vi "Call Remote Restart Camera server.vi"() -> (0 "Error out":errorcluster)   [LabVIEW 2015]
doc: "Asynchronously gets a snapshot image from the selected camera on the camera server and saves it to the specified path with specified name."
panel:
  # "PN 08/08/16"
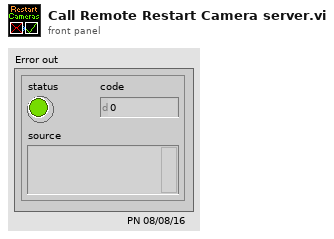
[diagram p1: front panel]
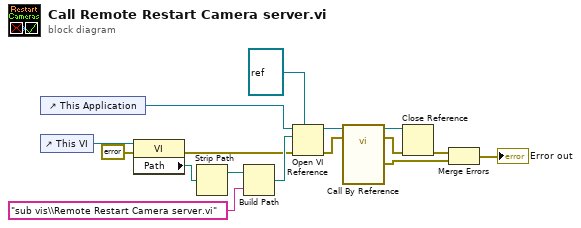
[diagram p0: block diagram]
diagram:
  n1 = control-ref of="This Application"() -> (w11:refnum<vi>)
  n2 = control-ref of="This VI"() -> (w16:refnum<vi>)
  n3 = property class="VI"(reference=w16, error in=errorcluster {"status"=FALSE, "code"=0, "source"=""} ("error in (no error)")) -> (error out=w13:errorcluster, "Path"=w10:path)  [unwired: 1 out]
  n4 = Strip Path(path=w10) -> (stripped path=w9:path)  [unwired: 1 out]
  n5 = Build Path(base path=w9, name or relative path="sub vis\\Remote Restart Camera server.vi") -> (appended path=w14:path)
  n6 = Open VI Reference(type specifier VI Refnum (for type only)=refnum<vi> refnum, application reference (local)=w11, vi path=w14, error in (no error)=w13) -> (vi reference=w8:refnum<vi>, error out=w7:errorcluster)  [unwired: 2 in]
  n7 = call-by-ref "?"(reference=w8, error in=w7) -> (reference out=w3:refnum<vi>, error out=w2:errorcluster, "Error out"=w1:errorcluster)
  n8 = Close Reference(reference=w3, error in (no error)=w2) -> (error out=w6:errorcluster)
  n9 = Merge Errors(w6, w1) -> (→"Error out":errorcluster)
